vi "UDP message to Data Log Strings.vi"(4 "Values":string[](array[string]), 5 "UUIDs":string[](array[string])) -> (0 "Data String":string, 1 "Header String":string)   [LabVIEW 2020]
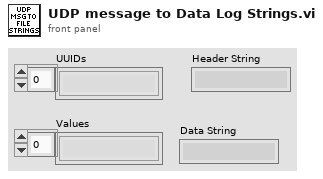
[diagram p1: front panel]
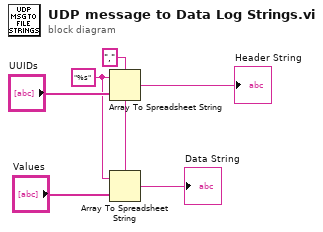
[diagram p0: block diagram]
diagram:
  w5 = "%s" ("format string")
  w1 = ","
  n1 = Array To Spreadsheet String(delimiter (Tab)=w1, array="UUIDs", 3:w5) -> (spreadsheet string=→"Header String":string)
  n2 = Array To Spreadsheet String(delimiter (Tab)=w1, array="Values", 3:w5) -> (spreadsheet string=→"Data String":string)
